vi "initUART.vi"(8 "error in (no error)":errorcluster, 11 "GiaoTiep in":refnum<class "GiaoTiepUART.lvclass">) -> (0 "error out":errorcluster, 3 "GiaoTiep out":refnum<class "GiaoTiepUART.lvclass">)   [LabVIEW 2014, in "LibraryGcode.lvlib" / "GiaoTiepUART.lvclass"]
uses:
  GiaoTiepUART.lvclass
  GiaoTiepUART.lvclass/GiaoTiepUART.ctl
  <vilib>/Instr/_visa.llb/VISA Configure Serial Port (Instr).vi
panel:
  in  "termination char\n(0xA = '\\n' = LF)":u8=10 format="%.0x"
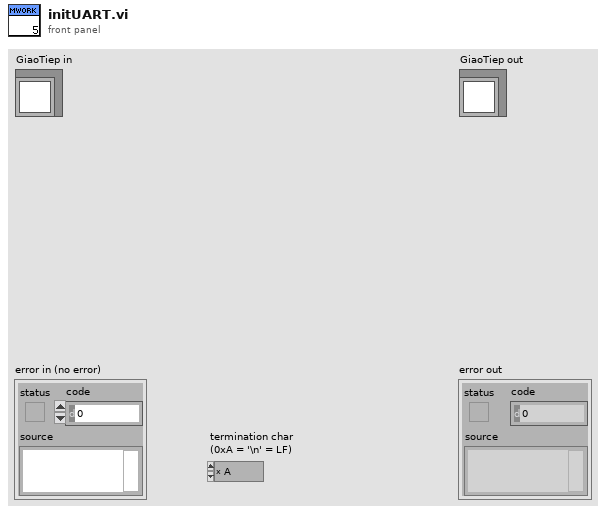
[diagram p1: front panel]
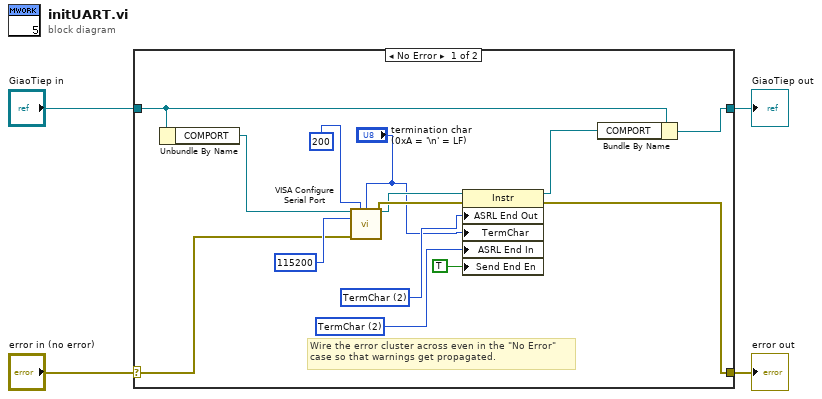
[diagram p0: block diagram]
diagram:
  n1 = case shown="No Error" "error in (no error)" {
    selector: "error in (no error)" -> [w10 w20]
    tunnel: [w9 w20] -> w3
    tunnel: [w6 w19] -> w1
    tunnel: "GiaoTiep in" -> [w7 w19]
    frame No Error {
      w12 = u16 2 items=["None", "Last Bit", "TermChar"] ("Serial Settings:End Mode for Reads")
      w17 = u16 2 items=["None", "Last Bit", "TermChar", "Break"] ("Serial Settings:End Mode for Writes")
      # "Wire the error cluster across even in the \"No Error\"\ncase so that warnings get propagated."
      n2 = Unbundle By Name(w7) -> ("COMPORT"=w8:refnum<visa-resource-name>)
      n3 = call-poly "VISA Configure Serial Port"("VISA resource name"=w8, "timeout (10sec)"=u32 200, "termination char\n(0xA = '\\n' = LF)"="termination char\n(0xA = '\\n' = LF)", "baud rate (9600)"=u32 115200, "error in (no error)"=w10) -> ("VISA resource name out"=w14:refnum<visa-resource-name>, "error out"=w15:errorcluster)  [unwired: 9 in]
      n4 = property class="Instr"(reference=w14, error in=w15, "ASRL End Out"=w17, "TermChar"="termination char\n(0xA = '\\n' = LF)", "ASRL End In"=w12, "Send End En"=TRUE ("Message Based Settings:Send End Enable")) -> (reference out=w5:refnum<visa-resource-name>, error out=w9:errorcluster)
      n5 = Bundle By Name(cluster=w7, "COMPORT"=w5) -> (w6:refnum<class "GiaoTiepUART.lvclass">)
    }
    frame Error {
    }
  }
  "error out" <- w3
  "GiaoTiep out" <- w1
